vi "Main.vi"() -> ()   [LabVIEW 2017]
doc: "Use this template to build a simple state machine design pattern. Each state executes code and determines which state to transition to."
uses:
  controls/State.ctl
  controls/Keithley input.ctl
  C:/Users/Biorgel/Documents/HZ/Bias PL/Thorlabs.MotionControl.Controls.dll
  Thorlabs.MotionControl.Controls.dll
  <instrlib>/Keithley 24XX/Keithley 24XX.lvlib
panel:
  out "Current Response (A)":dbl[][](array[numeric]) format="%#_3g"
  in  "Voltage Bias Output (V)":dbl[](array[numeric]) min=-36.0 max=36.0 step=0.001
  in  "Apply the previous voltage":bool
  in  "Keithley Address":refnum<visa-resource-name>="GPIB0::25::INSTR"
  in  "FilterFlipperControl":refnum<k24>(container)
  in  "Apply the current voltage":bool
  in  "Apply the next votlage":bool
  in  "Exit":bool
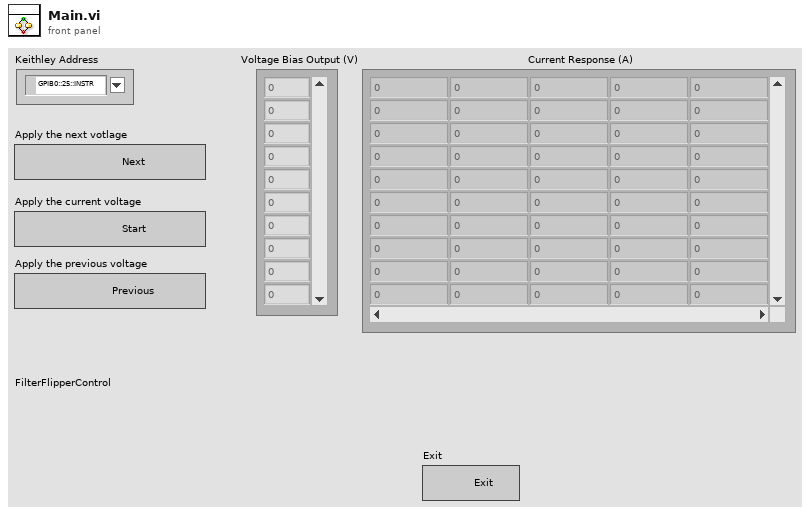
[diagram p1: front panel]
types:
  T1 = typedef "Keithley input.ctl" = cluster{"Sample Count (10)":i32, "Timeout (10000 ms)":i32, "Compliance  Level (0.1)":dbl, "Output Level (0)":dbl, "Source Mode  (0: Voltage)":u16, "Output sequence":i32, "Output list":dbl[]}
  T2 = typedef "State.ctl" = enum16{"Initialize", "Wait for Event", "State 1 apply bias", "State2 this bias", "State3 previous bias", "output on", "Exit"}
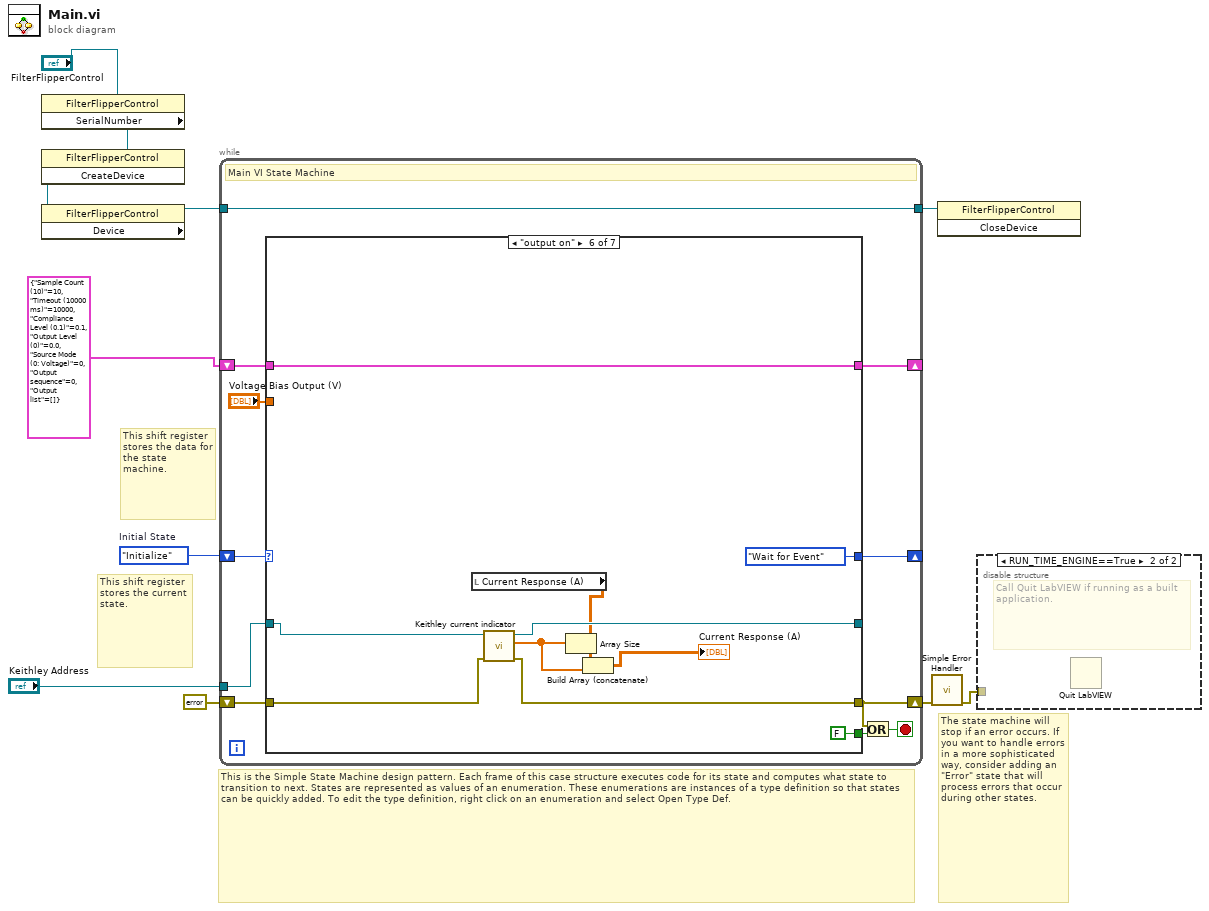
[diagram p0: block diagram]
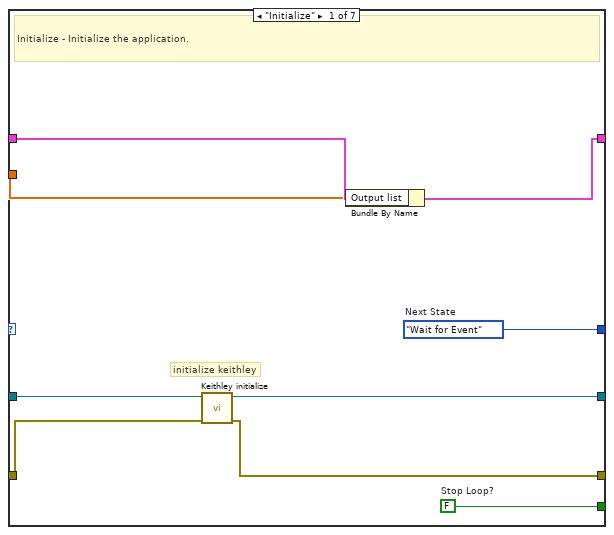
[diagram p3: hidden frame]
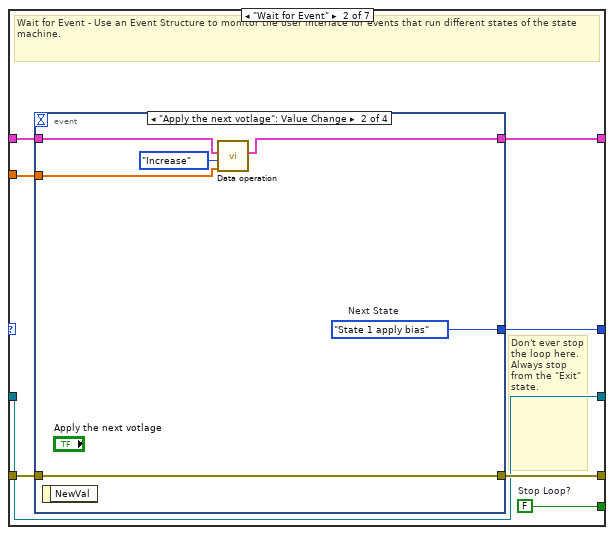
[diagram p4: hidden frame]
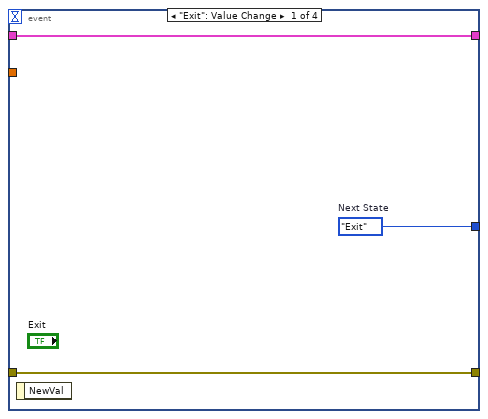
[diagram p5: hidden frame]
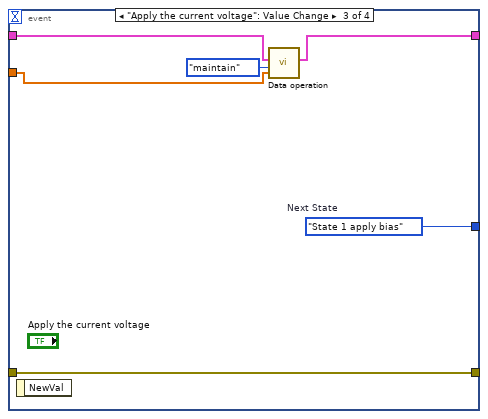
[diagram p6: hidden frame]
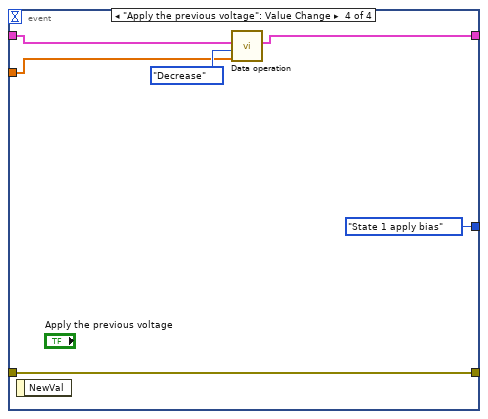
[diagram p7: hidden frame]
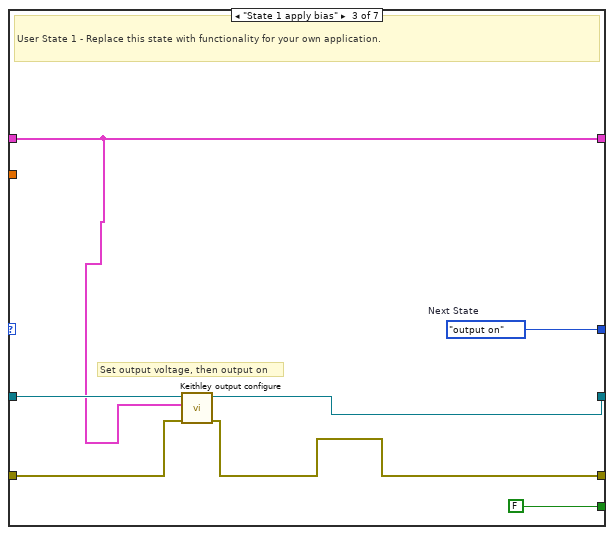
[diagram p8: hidden frame]
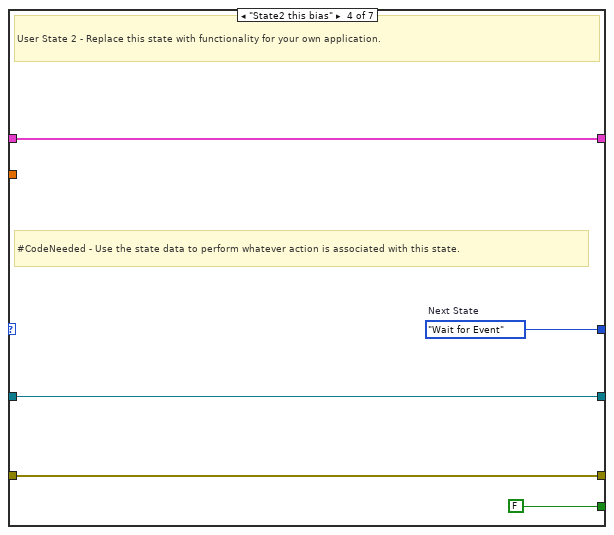
[diagram p9: hidden frame]
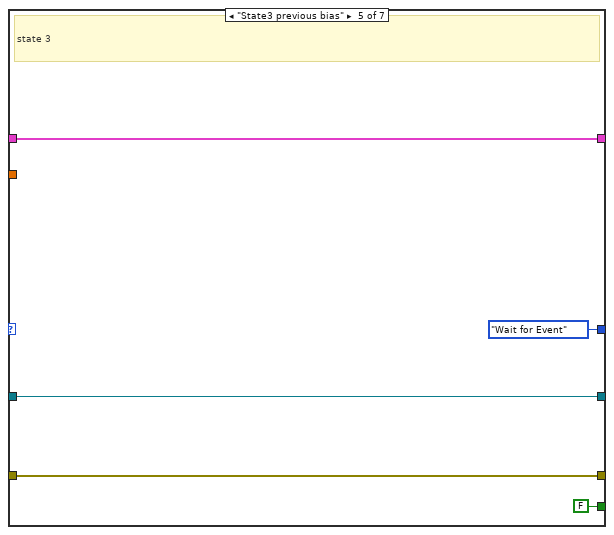
[diagram p10: hidden frame]
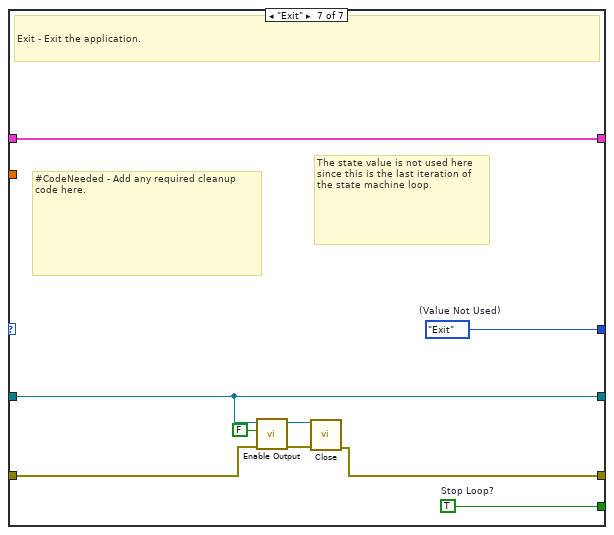
[diagram p11: hidden frame]
diagram:
  w11 = State."Initialize"  # Initial State
  # "The state machine will stop if an error occurs. If you want to handle errors in a more sophisticated way, consider adding an \"Error\" state that will process errors that occur during other states."
  # "This shift register stores the data for the state machine."
  # "This is the Simple State Machine design pattern. Each frame of this case structure executes code for its state and computes what state to transition to next. States are represented as values of an enumeration. These enumerations are instances of a type definition so that states can be quickly added. To edit the type definition, right click on an enumeration and select Open Type Def."
  # "This shift register stores the current state."
  n1 = property class="FilterFlipperControl" props=["SerialNumber"](reference="FilterFlipperControl") -> (reference out=w7:refnum<k24>)  [unwired: 1 in, 2 out]
  n2 = invoke class="FilterFlipperControl" method="CreateDevice"(reference=w7) -> (reference out=w6:refnum<k24>)  [unwired: 2 in, 2 out]
  n3 = property class="FilterFlipperControl" props=["Device"](reference=w6) -> (reference out=w5:refnum<k24>)  [unwired: 1 in, 2 out]
  n4 = while {
    shift-right: [w21] -> _
    shift-left: w11 -> [w22]
    shift-right: [w19] -> _
    shift-left: T1 {"Sample Count (10)"=10, "Timeout (10000 ms)"=10000, "Compliance  Level (0.1)"=0.1, "Output Level (0)"=0.0, "Source Mode  (0: Voltage)"=0, "Output sequence"=0, "Output list"=[]} ("Keithley Output Configure") -> [w20]
    shift-right: [w15] -> w9
    shift-left: errorcluster {"status"=FALSE, "code"=0, "source"=""} ("error constant") -> [w18]
    tunnel: w5 -> [w14]
    tunnel: [w14] -> w4
    tunnel: "Keithley Address" -> [w13]
    stop <- w16 stop-if-true
    # "Main VI State Machine"
    n5 = case shown="\"output on\"" w22 {
      tunnel: [w31 w39 w67 w72 State."Wait for Event" ("(Value Not Used)") State."Wait for Event" ("(Value Not Used)") w96] -> w21
      tunnel: [w30 w38 FALSE ("Stop Loop?") FALSE ("Stop Loop?") FALSE ("Stop Loop?") FALSE ("Stop Loop?") w94] -> w17
      tunnel: w20 -> [w25 w37 w61 w70 w77 w87 w95]
      tunnel: [w24 w36 w61 w70 w77 w87 w95] -> w19
      tunnel: w18 -> [w27 w35 w64 w68 w76 w83 w91]
      tunnel: [w26 w34 w62 w68 w76 w82 w88] -> w15
      tunnel: [w28 w33 w63 w69 w73 w84 w93] -> _
      tunnel: w13 -> [w29 w33 w65 w69 w73 w85 w93]
      tunnel: "Voltage Bias Output (V)" -> [w23 w32 _ _ _ _ _]
      frame "Initialize" {
        w30 = FALSE  # Stop Loop?
        w31 = State."Wait for Event"  # Next State
        # "initialize keithley"
        # "Initialize - Initialize the application."
        n6 = call "Keithley initialize.vi"("error in (no error)"=w27, "VISA resource name"=w29) -> ("error out"=w26:errorcluster, "VISA resource name out"=w28:refnum<visa-resource-name>)  [unwired: 8 in]
        n7 = Bundle By Name(cluster=w25, "Output list"=w23) -> (w24:T1)
      }
      frame "Wait for Event" {
        w38 = FALSE  # Stop Loop?
        # "Don't ever stop the loop here. Always stop from the \"Exit\" state."
        # "Wait for Event - Use an Event Structure to monitor the user interface for events that run different states of the state machine."
        n8 = event shown="[1] \"Apply the next votlage\": Value Change" {
          selector: _ -> [_ _ _ _]
          dyn-events: _ -> [_ _ _ _]
          timeout: _ -> [_ _ _ _]
          tunnel: [w42 w48 w54 State."State 1 apply bias" ("Next State")] -> w39
          tunnel: w37 -> [w41 w46 w51 w57]
          tunnel: [w41 w45 w50 w56] -> w36
          tunnel: w35 -> [w40 w47 w53 w60]
          tunnel: [w40 w47 w53 w60] -> w34
          tunnel: w32 -> [_ w43 w49 w55]
          event "Exit": Value Change {
            w42 = State."Exit"  # Next State
            n9 = event-data() -> ()  [unwired: 1 in, 1 out]
          }
          event "Apply the next votlage": Value Change {
            w48 = State."State 1 apply bias"  # Next State
            n10 = event-data() -> ()  [unwired: 1 in, 1 out]
            n11 = call "Data operation.vi"("Output list"=w43, "Operation"=enum16{"Increase", "maintain", "Decrease"}."Increase", "Keithley Output Configure"=w46) -> ("Keithley Output Configure 2"=w45:T1)  [unwired: 8 in]
          }
          event "Apply the current voltage": Value Change {
            w54 = State."State 1 apply bias"  # Next State
            n12 = event-data() -> ()  [unwired: 1 in, 1 out]
            n13 = call "Data operation.vi"("Output list"=w49, "Operation"=enum16{"Increase", "maintain", "Decrease"}."maintain", "Keithley Output Configure"=w51) -> ("Keithley Output Configure 2"=w50:T1)  [unwired: 8 in]
          }
          event "Apply the previous voltage": Value Change {
            n14 = event-data() -> ()  [unwired: 1 in, 1 out]
            n15 = call "Data operation.vi"("Output list"=w55, "Operation"=enum16{"Increase", "maintain", "Decrease"}."Decrease", "Keithley Output Configure"=w57) -> ("Keithley Output Configure 2"=w56:T1)  [unwired: 8 in]
          }
        }
      }
      frame "State 1 apply bias" {
        w67 = State."output on"  # Next State
        # "Set output voltage, then output on"
        # "User State 1 - Replace this state with functionality for your own application."
        n16 = call "Keithley output configure.vi"("error in (no error)"=w64, "Keithley Output Configure"=w61, "VISA resource name"=w65) -> ("error out"=w62:errorcluster, "VISA resource name out"=w63:refnum<visa-resource-name>)  [unwired: 7 in]
      }
      frame "State2 this bias" {
        w72 = State."Wait for Event"  # Next State
        # "#CodeNeeded - Use the state data to perform whatever action is associated with this state."
        # "User State 2 - Replace this state with functionality for your own application."
      }
      frame "State3 previous bias" {
        # "state 3"
      }
      frame "output on" {
        n17 = local read "Current Response (A)"() -> (w78:dbl[][])
        n18 = call "Keithley current indicator.vi"("error in (no error)"=w83, "VISA resource name"=w85) -> ("error out"=w82:errorcluster, "appended array"=w81:sgl[], "VISA resource name out"=w84:refnum<visa-resource-name>)  [unwired: 7 in]
        n19 = Array Size(array=w81) -> ()  [unwired: 1 out]
        n20 = Build Array (concatenate)(w78, w81) -> (→"Current Response (A)":dbl[][])
      }
      frame "Exit" {
        w94 = TRUE  # Stop Loop?
        w96 = State."Exit"  # (Value Not Used)
        # "#CodeNeeded - Add any required cleanup code here."
        # "The state value is not used here since this is the last iteration of the state machine loop."
        # "Exit - Exit the application."
        n21 = call <instrlib>:"Enable Output.vi"("error in (no error)"=w91, "Enable Output (T: Enable)"=FALSE, "VISA resource name"=w93) -> ("error out"=w90:errorcluster, "VISA resource name out"=w89:refnum<visa-resource-name>)  [unwired: 7 in]
        n22 = call <instrlib>:"Close.vi"("error in (no error)"=w90, "VISA resource name"=w89) -> ("error out"=w88:errorcluster)  [unwired: 9 in]
      }
    }
    n23 = Or(x=w15, y=w17) -> (x .or. y?=w16:bool)
  }
  n24 = call <vilib>:"Simple Error Handler.vi"("error in (no error)"=w9) -> ("error out"=w8:errorcluster)  [unwired: 4 in, 4 out]
  n25 = invoke class="FilterFlipperControl" method="CloseDevice"(reference=w4) -> ()  [unwired: 2 in, 3 out]
  n26 = disable-structure shown="RUN_TIME_ENGINE==True" {
    disable-tunnel: w8 -> [_ _]
    frame condition #0 (active) {
    }
    frame condition #1 {
      # "Call Quit LabVIEW if running as a built application."
      n27 = Quit LabVIEW() -> ()  [unwired: 1 in]
    }
  }
